vi "getStyleByName.vi"(8 "error in (no error)":errorcluster, 10 "Style Name":string, 11 "MS-Excel in":refnum<class "MS-Excel.lvclass">) -> (0 "error out":errorcluster, 2 "Style":variant, 3 "MS-Excel out":refnum<class "MS-Excel.lvclass">)   [LabVIEW 2020, in "LabVIEW NPOI.lvlib" / "MS-Excel.lvclass"]
uses:
  MS-Excel.lvclass
  Document/Document.lvclass
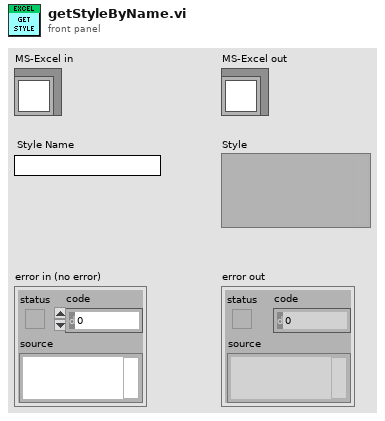
[diagram p1: front panel]
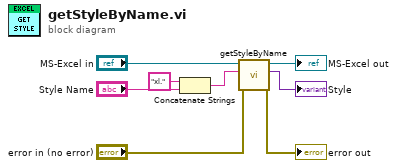
[diagram p0: block diagram]
diagram:
  n1 = Concatenate Strings("xl." ("string"), "Style Name") -> (w2:string)
  n2 = call-parent "getStyleByName.vi"("error in (no error)"="error in (no error)", "Style Name"=w2, "Document in"="MS-Excel in") -> ("error out"=→"error out":errorcluster, "Style"=→"Style":variant, "Document out"=→"MS-Excel out":refnum<class "MS-Excel.lvclass">)  [unwired: 6 in]
